vi "snappinginloop.vi"() -> ()   [LabVIEW 2009]
uses:
  <vilib>/vision/NI_Vision_Development_Module.lvlib
panel:
  in  "stop":bool
  out "Live saturation image":T1(plugin-control)
  out "Live image":T1(plugin-control)
  out "Histogram graph 3":T2(graph)
  in  "ON":bool
  out "?":string
  out "?":string
  in  "Custom snapshot":bool
  in  "BF snapshot":bool
  in  "RFP snapshot":bool
  in  "YFP snapshot":bool
  in  "GFP snapshot":bool
  in  "Red snapshot":bool
  in  "Green snapshot":bool
  in  "Manual or automatic":bool
  in  "Read path automatically from:":path
  out "Data path label":string
  out "Directory":string
  in  "Save path":path
  in  "Panel label":string
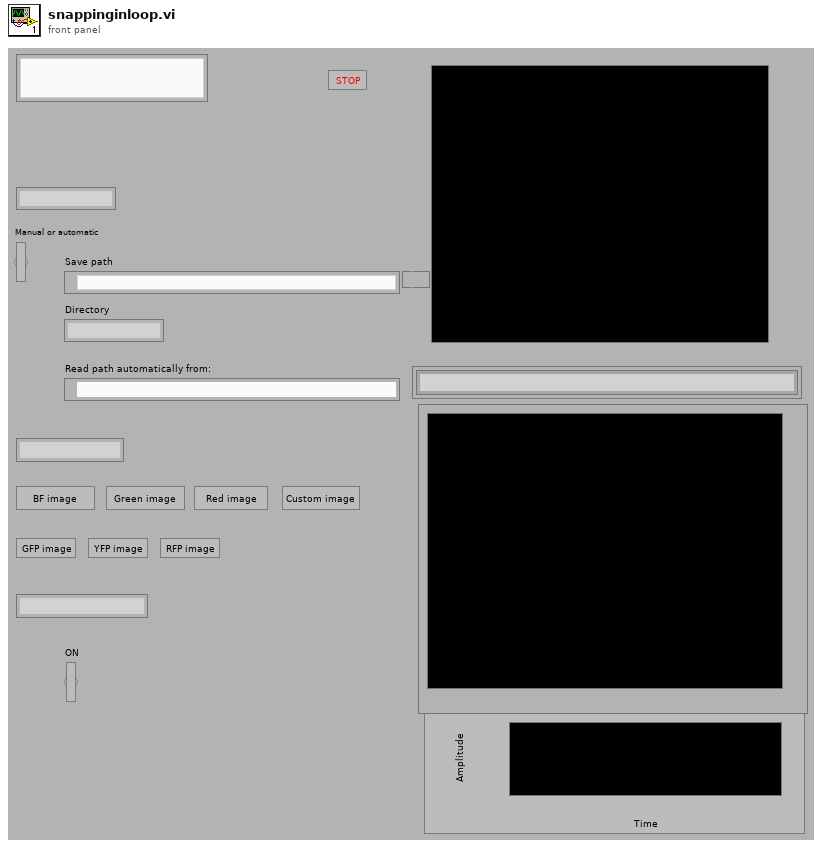
[diagram p1: front panel]
types:
  T1 = typedef "IMAQ Image.ctl" = refnum<image>
  T2 = cluster{"Starting Value":sgl, "Incremental Value":sgl, "Histogram":u32[]}
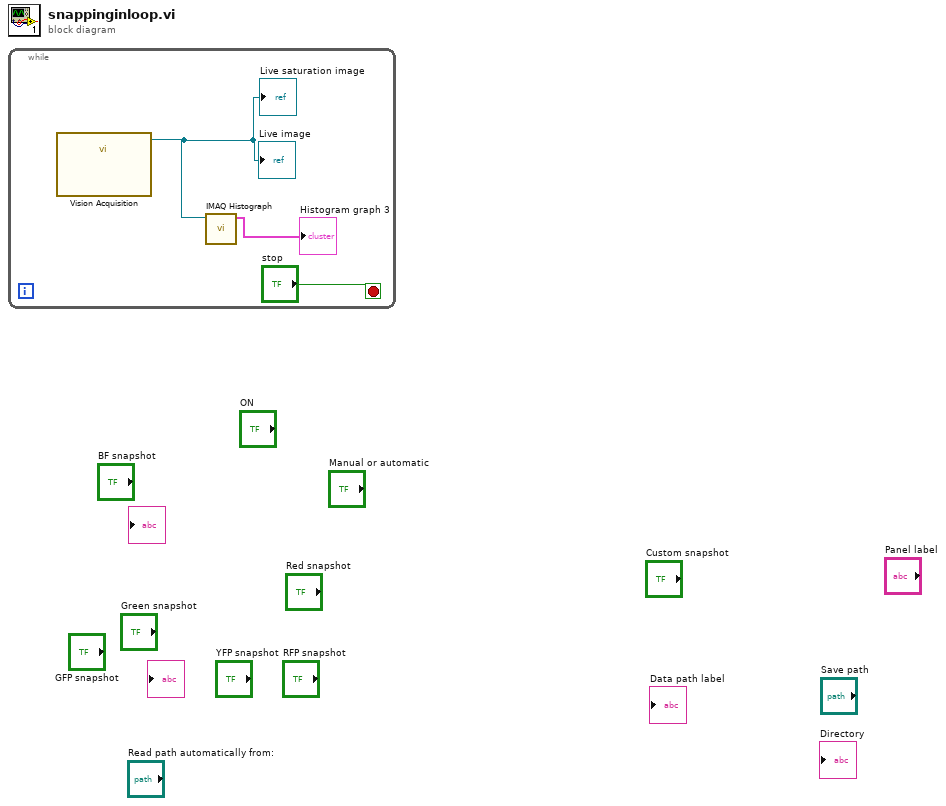
[diagram p0: block diagram]
diagram:
  n1 = while {
    stop <- "stop" stop-if-true
    n2 = call "Vision Acquisition"() -> ("Image Out"=w2:T1)  [unwired: 26 in, 1 out]
    "Live saturation image" <- w2
    "Live image" <- w2
    n3 = call "IMAQ Histograph"("Image"=w2) -> ("Histogram Graph"=→"Histogram graph 3":T2)  [unwired: 7 in, 3 out]
  }
